vi "Kiwi_Open.vi"(6 "MotorInverters":T11, 7 "Angles":T1={"Angle A"=60.0, "Angle B"=60.0, "Angle C"=60.0}, 8 "Device Channels":T3, 9 "MotorType":enum16{"CAN SRX", "PWM SRX", "SR"}(ring), 10 "RefnumName":string, 11 "MotorDevRefsIn":T4={"Motor A"={"DeviceStatus"={"status"=FALSE, "code"=0, "source"=""}, "Type"=enum."PWM", "PWM"={"PWM Channel"=enum."Invalid", "DeadBand"={"Name"="", "maxPositivePwm"=0, "minPositivePwm"=0, "centerPwm"=0, "maxNegativePwm"=0, "minNegativePwm"=0, "angularRange"=0}}, "CAN"={"Device Number"=0, "Control Mode"=enum."Percent VBus", "Semaphore"=refnum, "Max Vout"=12.0, "TalonSRX Control Mode"=enum."Percent VBus"}, "Invert"=FALSE}, "Motor B"={"DeviceStatus"={"status"=FALSE, "code"=0, "source"=""}, "Type"=enum."PWM", "PWM"={"PWM Channel"=enum."Invalid", "DeadBand"={"Name"="", "maxPositivePwm"=0, "minPositivePwm"=0, "centerPwm"=0, "maxNegativePwm"=0, "minNegativePwm"=0, "angularRange"=0}}, "CAN"={"Device Number"=0, "Control Mode"=enum."Percent VBus", "Semaphore"=refnum, "Max Vout"=12.0, "TalonSRX Control Mode"=enum."Percent VBus"}, "Invert"=FALSE}, "Motor C"={"DeviceStatus"={"status"=FALSE, "code"=0, "source"=""}, "Type"=enum."PWM", "PWM"={"PWM Channel"=enum."Invalid", "DeadBand"={"Name"="", "maxPositivePwm"=0, "minPositivePwm"=0, "centerPwm"=0, "maxNegativePwm"=0, "minNegativePwm"=0, "angularRange"=0}}, "CAN"={"Device Number"=0, "Control Mode"=enum."Percent VBus", "Semaphore"=refnum, "Max Vout"=12.0, "TalonSRX Control Mode"=enum."Percent VBus"}, "Invert"=FALSE}, "Config Consts"={"Constant One"=0.0, "Constant Two"=0.0, "Constant Three"=0.0, "Constant Four"=0.0, "Constant FIve"=0.0, "Constant Six"=0.0}}) -> (3 "MotorDevRefsOut":T4={"Motor A"={"DeviceStatus"={"status"=FALSE, "code"=0, "source"=""}, "Type"=enum."PWM", "PWM"={"PWM Channel"=enum."Invalid", "DeadBand"={"Name"="", "maxPositivePwm"=0, "minPositivePwm"=0, "centerPwm"=0, "maxNegativePwm"=0, "minNegativePwm"=0, "angularRange"=0}}, "CAN"={"Device Number"=0, "Control Mode"=enum."Percent VBus", "Semaphore"=refnum, "Max Vout"=12.0, "TalonSRX Control Mode"=enum."Percent VBus"}, "Invert"=FALSE}, "Motor B"={"DeviceStatus"={"status"=FALSE, "code"=0, "source"=""}, "Type"=enum."PWM", "PWM"={"PWM Channel"=enum."Invalid", "DeadBand"={"Name"="", "maxPositivePwm"=0, "minPositivePwm"=0, "centerPwm"=0, "maxNegativePwm"=0, "minNegativePwm"=0, "angularRange"=0}}, "CAN"={"Device Number"=0, "Control Mode"=enum."Percent VBus", "Semaphore"=refnum, "Max Vout"=12.0, "TalonSRX Control Mode"=enum."Percent VBus"}, "Invert"=FALSE}, "Motor C"={"DeviceStatus"={"status"=FALSE, "code"=0, "source"=""}, "Type"=enum."PWM", "PWM"={"PWM Channel"=enum."Invalid", "DeadBand"={"Name"="", "maxPositivePwm"=0, "minPositivePwm"=0, "centerPwm"=0, "maxNegativePwm"=0, "minNegativePwm"=0, "angularRange"=0}}, "CAN"={"Device Number"=0, "Control Mode"=enum."Percent VBus", "Semaphore"=refnum, "Max Vout"=12.0, "TalonSRX Control Mode"=enum."Percent VBus"}, "Invert"=FALSE}, "Config Consts"={"Constant One"=0.0, "Constant Two"=0.0, "Constant Three"=0.0, "Constant Four"=0.0, "Constant FIve"=0.0, "Constant Six"=0.0}})   [LabVIEW 2015]
uses:
  <userlib>/836-Library/Drive/kiwi/Kiwi_Dev_Ref.ctl
  <vilib>/Rock Robotics/WPI/MotorControl/WPI_MotorControlDeviceRef.ctl
  <vilib>/Rock Robotics/WPI/MotorControl/WPI_MotorControlType.ctl
  <vilib>/Rock Robotics/SystemInterfaces/DIO/FPGA_DIOPWMChannel.ctl
  <vilib>/Rock Robotics/WPI/PWM/WPI_PWMDeadband.ctl
  <vilib>/Rock Robotics/WPI/CAN/Jaguar/SubVIs/WPI_CANJaguar_ControlMode.ctl
  <vilib>/Rock Robotics/WPI/CAN/TalonSRX/WPI_CANTalonSRX_APIControlMode.ctl
  <vilib>/Rock Robotics/WPI/Utilities/Refnum Registry Operation.ctl
  <vilib>/Rock Robotics/WPI/MotorControl/WPI_MotorControlOpenCANTalonSRX.vi
  <vilib>/Rock Robotics/WPI/MotorControl/WPI_MotorControlOpen TalonSRX.vi
  <vilib>/Rock Robotics/WPI/MotorControl/WPI_MotorControlOpen Talon.vi
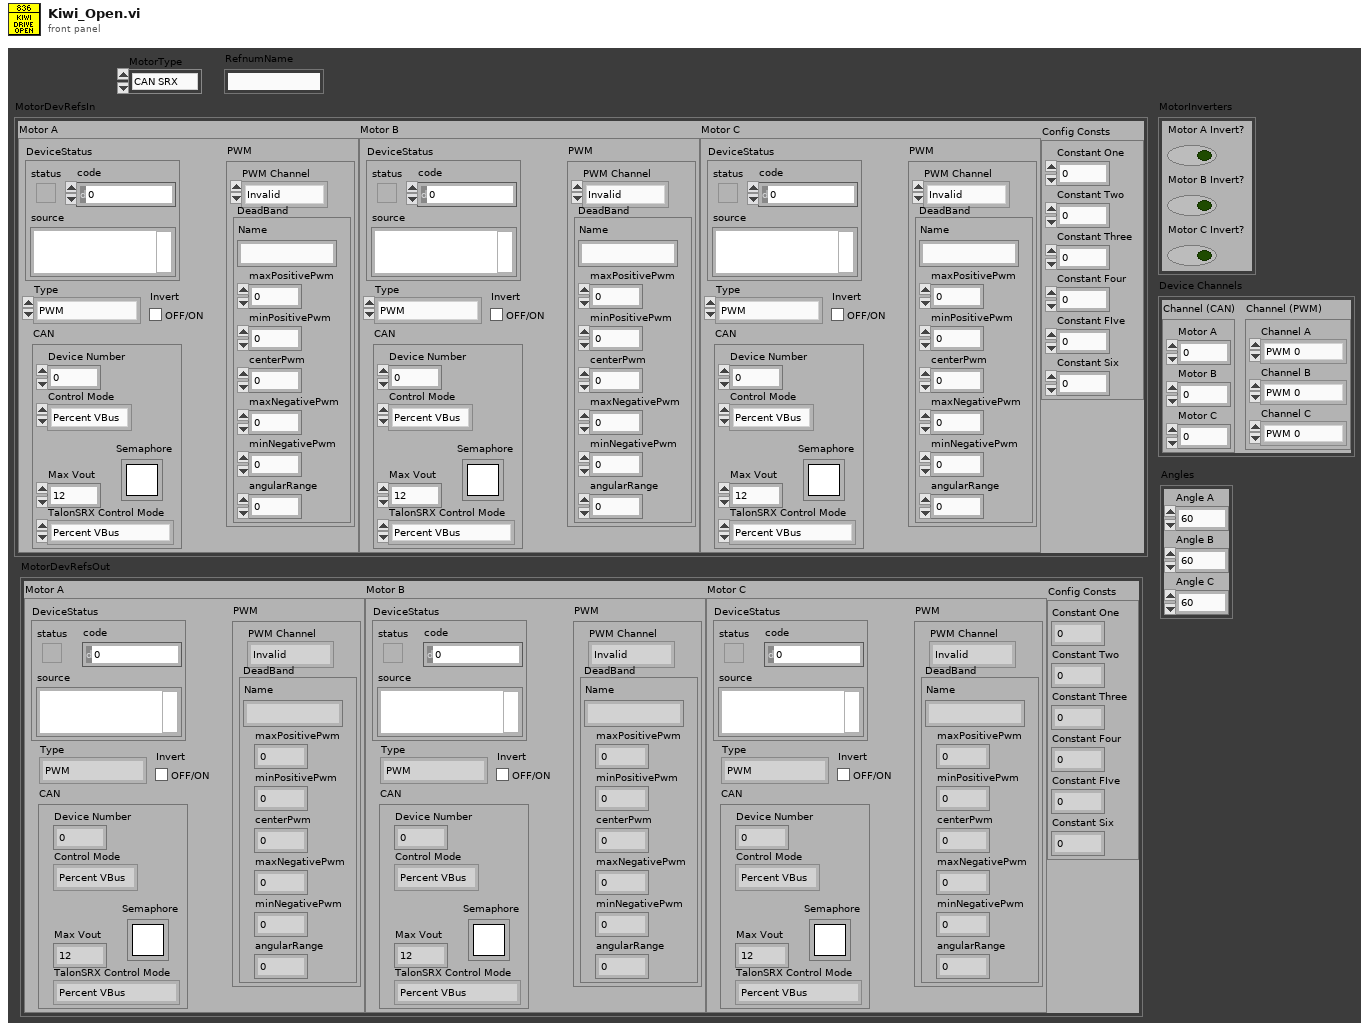
[diagram p1: front panel]
types:
  T1 = cluster{"Angle A":dbl, "Angle B":dbl, "Angle C":dbl}
  T2 = typedef "FPGA_DIOPWMChannel.ctl" = enum8{"PWM 0", "PWM 1", "PWM 2", "PWM 3", "PWM 4", "PWM 5", "PWM 6", "PWM 7", "PWM 8", "PWM 9", "PWM MXP 0", "PWM MXP 1", "PWM MXP 2", "PWM MXP 3", "PWM MXP 4", "PWM MXP 5", "PWM MXP 6", "PWM MXP 7", "PWM MXP 8", "PWM MXP 9", "Invalid"}
  T3 = cluster{"Channel (CAN)":cluster{"Motor A":u8, "Motor B":u8, "Motor C":u8}, "Channel (PWM)":cluster{"Channel A":T2, "Channel B":T2, "Channel C":T2}}
  T4 = typedef "Kiwi_Dev_Ref.ctl" = cluster{"Motor A":T5, "Motor B":T5, "Motor C":T5, "Config Consts":cluster{"Constant One":dbl, "Constant Two":dbl, "Constant Three":dbl, "Constant Four":dbl, "Constant FIve":dbl, "Constant Six":dbl}}
  T5 = typedef "WPI_MotorControlDeviceRef.ctl" = cluster{"DeviceStatus":errorcluster, "Type":T6, "PWM":cluster{"PWM Channel":T2, "DeadBand":T7}, "CAN":cluster{"Device Number":u8, "Control Mode":T8, "Semaphore":T9, "Max Vout":dbl, "TalonSRX Control Mode":T10}, "Invert":bool}
  T6 = typedef "WPI_MotorControlType.ctl" = enum16{"PWM", "CAN", "CANTalonSRX"}
  T7 = typedef "WPI_PWMDeadband.ctl" = cluster{"Name":string, "maxPositivePwm":i32, "minPositivePwm":i32, "centerPwm":i32, "maxNegativePwm":i32, "minNegativePwm":i32, "angularRange":u16}
  T8 = typedef "WPI_CANJaguar_ControlMode.ctl" = enum8{"Percent VBus", "Current", "Speed", "Position", "Voltage"}
  T9 = typedef "Semaphore RefNum" = refnum<k1>
  T10 = typedef "WPI_CANTalonSRX_APIControlMode.ctl" = enum8{"Percent VBus", "Speed", "Position", "Slave", "Unchanged / Invalid", "Voltage Compensation", "Current", "Motion Profile"}
  T11 = cluster{"Motor A Invert?":bool, "Motor B Invert?":bool, "Motor C Invert?":bool}
  T12 = typedef "Refnum Registry Operation.ctl" = enum16{"set", "get", "delete", "get all names", "read name"}
  T13 = cluster{"Motor A":u8, "Motor B":u8, "Motor C":u8}
  T14 = cluster{"Channel A":T2, "Channel B":T2, "Channel C":T2}
  T15 = cluster{"Constant One":dbl, "Constnat Two":dbl, "Consnat Three":dbl, "Constant Four":dbl, "Constant Five":dbl, "Constant Six":dbl}
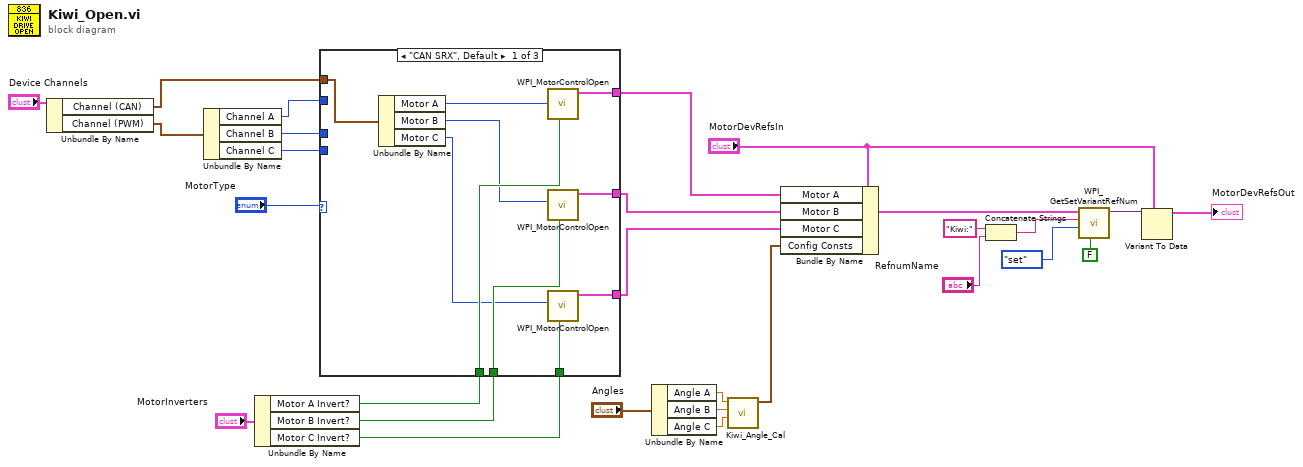
[diagram p0: block diagram]
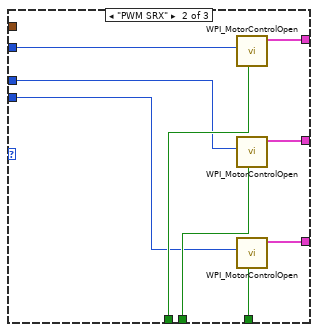
[diagram p2: hidden frame]
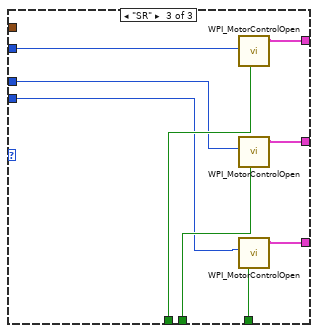
[diagram p3: hidden frame]
diagram:
  n1 = Unbundle By Name("Device Channels") -> ("Channel (CAN)"=w6:T13, "Channel (PWM)"=w7:T14)
  n2 = Unbundle By Name(w7) -> ("Channel A"=w11:T2, "Channel B"=w10:T2, "Channel C"=w9:T2)
  n3 = Unbundle By Name("MotorInverters") -> ("Motor A Invert?"=w21:bool, "Motor B Invert?"=w22:bool, "Motor C Invert?"=w23:bool)
  n4 = case shown="\"CAN SRX\", Default" "MotorType" {
    tunnel: [w38 w47 w56] -> w27
    tunnel: [w37 w46 w55] -> w26
    tunnel: [w36 w45 w54] -> w25
    tunnel: w23 -> [w35 w44 w53]
    tunnel: w22 -> [w34 w43 w52]
    tunnel: w21 -> [w33 w42 w51]
    tunnel: w11 -> [_ w41 w50]
    tunnel: w10 -> [_ w40 w49]
    tunnel: w9 -> [_ w39 w48]
    tunnel: w6 -> [w29 _ _]
    frame "CAN SRX", Default {
      n5 = Unbundle By Name(w29) -> ("Motor A"=w32:u8, "Motor B"=w31:u8, "Motor C"=w30:u8)
      n6 = call-poly <vilib>:"WPI_MotorControlOpen.vi"("Invert"=w33, "Device Number"=w32) -> ("MotorControlDeviceRef"=w38:T5)  [unwired: 8 in, 1 out]
      n7 = call-poly <vilib>:"WPI_MotorControlOpen.vi"("Invert"=w34, "Device Number"=w31) -> ("MotorControlDeviceRef"=w37:T5)  [unwired: 8 in, 1 out]
      n8 = call-poly <vilib>:"WPI_MotorControlOpen.vi"("Invert"=w35, "Device Number"=w30) -> ("MotorControlDeviceRef"=w36:T5)  [unwired: 8 in, 1 out]
    }
    frame "PWM SRX" {
      n9 = call-poly <vilib>:"WPI_MotorControlOpen.vi"("Invert"=w42, "PWM Channel"=w41) -> ("MotorControlDeviceRef"=w47:T5)  [unwired: 8 in, 1 out]
      n10 = call-poly <vilib>:"WPI_MotorControlOpen.vi"("Invert"=w43, "PWM Channel"=w40) -> ("MotorControlDeviceRef"=w46:T5)  [unwired: 8 in, 1 out]
      n11 = call-poly <vilib>:"WPI_MotorControlOpen.vi"("Invert"=w44, "PWM Channel"=w39) -> ("MotorControlDeviceRef"=w45:T5)  [unwired: 8 in, 1 out]
    }
    frame "SR" {
      n12 = call-poly <vilib>:"WPI_MotorControlOpen.vi"("Invert"=w51, "PWM Channel"=w50) -> ("MotorControlDeviceRef"=w56:T5)  [unwired: 8 in, 1 out]
      n13 = call-poly <vilib>:"WPI_MotorControlOpen.vi"("Invert"=w52, "PWM Channel"=w49) -> ("MotorControlDeviceRef"=w55:T5)  [unwired: 8 in, 1 out]
      n14 = call-poly <vilib>:"WPI_MotorControlOpen.vi"("Invert"=w53, "PWM Channel"=w48) -> ("MotorControlDeviceRef"=w54:T5)  [unwired: 8 in, 1 out]
    }
  }
  n15 = Unbundle By Name("Angles") -> ("Angle A"=w4:dbl, "Angle B"=w3:dbl, "Angle C"=w2:dbl)
  n16 = call <userlib>:"Kiwi_Angle_Cal.vi"("Angle C"=w2, "Angle B"=w3, "Angle A"=w4) -> ("Config Consts"=w1:T15)  [unwired: 8 in]
  n17 = Bundle By Name(cluster="MotorDevRefsIn", "Motor A"=w27, "Motor B"=w26, "Motor C"=w25, "Config Consts"=w1) -> (w20:T4)
  n18 = Concatenate Strings("Kiwi:" ("string"), "RefnumName") -> (w19:string)
  n19 = call <vilib>:"WPI_GetSetVariantRefNum.vi"("Test Mode Only"=FALSE, "Operation"=Refnum_Registry_Operation."set", "refnum name"=w19, "DevRef"=w20) -> ("DevRef"=w14:variant)  [unwired: 5 in, 2 out]
  n20 = Variant To Data(type="MotorDevRefsIn", Variant=w14) -> (data=→"MotorDevRefsOut":T4)  [unwired: 1 in, 1 out]
